vi "ReadChangedFileLogPaths.vi"(8 "error in (no error)":errorcluster, 10 "Workspace Path":path, 11 "Refnum in":T1) -> (0 "error out":errorcluster, 2 "ChangedFilesLogpaths":map{string, path}(c390), 3 "refnum out":T1)   [LabVIEW 2019, in "Hawkeye.lvlib"]
uses:
  Hawkeye.lvlib
  <vilib>/Utility/config.llb/Config Data RefNum.ctl
  <vilib>/Utility/config.llb/Read Key (String).vi
  <vilib>/Utility/config.llb/NI_LVConfig.lvlib
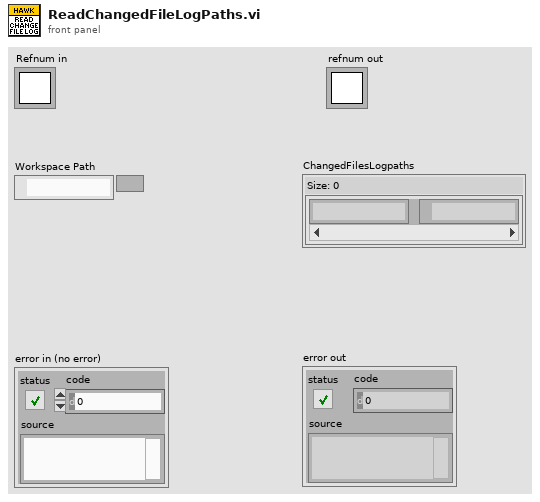
[diagram p1: front panel]
types:
  T1 = typedef "NI_LVConfig.lvlib/Config Data RefNum.ctl" = refnum<k1>
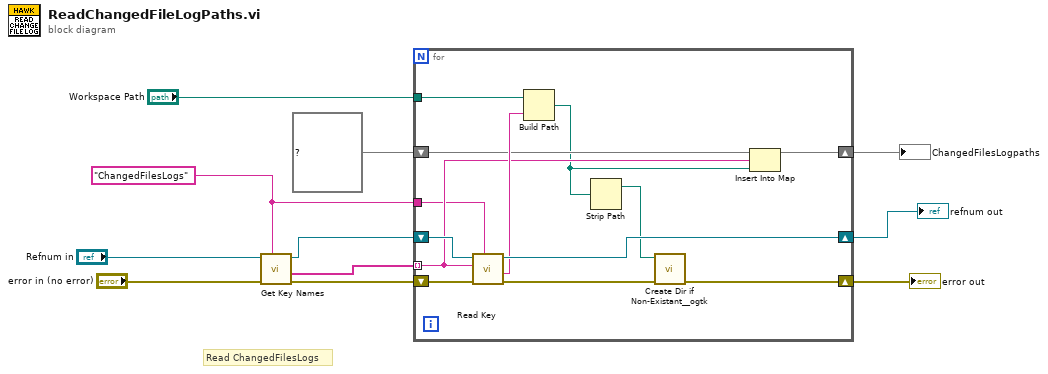
[diagram p0: block diagram]
diagram:
  w1 = "ChangedFilesLogs" ("section")
  # "Read ChangedFilesLogs"
  n1 = call <vilib>:"Get Key Names.vi"("section"=w1, "error in (no error)"="error in (no error)", "refnum"="Refnum in") -> ("error out"=w9:errorcluster, "key names"=w10:string[], "refnum out"=w8:T1)  [unwired: 5 in, 1 out]
  n2 = for {
    shift-right: [w16] -> w4
    shift-left: w9 -> [w12]
    tunnel: w10 -> [w19] mode=indexing
    tunnel: "Workspace Path" -> [w24]
    shift-right: [w22] -> w5
    shift-left: w8 -> [w23]
    shift-right: [w18] -> w2
    shift-left: map{string, path} {} ("map") -> [w20]
    tunnel: w1 -> [w17]
    n3 = call-poly <vilib>:"Read Key.vi"("section"=w17, "error in (no error)"=w12, "key"=w19, "refnum"=w23) -> ("error out"=w13:errorcluster, "value"=w21:string, "refnum out"=w22:T1)  [unwired: 4 in, 1 out]
    n4 = Build Path(base path=w24, name or relative path=w21) -> (appended path=w15:path)
    n5 = Strip Path(path=w15) -> (stripped path=w14:path)  [unwired: 1 out]
    n6 = call <userlib>:"Create Dir if Non-Existant__ogtk.vi"("error in (no error)"=w13, "Directory Path"=w14) -> ("error out"=w16:errorcluster)  [unwired: 7 in, 2 out]
    n7 = Insert Into Map(map in=w20, key=w19, value=w15) -> (map out=w18:map{string, path})  [unwired: 2 out]
  }
  "refnum out" <- w5
  "error out" <- w4
  "ChangedFilesLogpaths" <- w2
